vi "SetAutomaticParameterMode.vi"(7 "Auto Parameter":T2, 8 "error in (no error)":errorcluster, 10 "Automatic":T1, 11 "Stream in":refnum<class "Stream.lvclass">) -> (0 "error out":errorcluster, 3 "Stream (Duplicate)":refnum<class "Stream.lvclass">)   [LabVIEW 2020, in "g_ar_toolkit.capture.lvlib" / "Stream.lvclass"]
uses:
  Stream.lvclass
  Camera Automatic Parameters.ctl
  Camera Automatic Parameter Mode.ctl
  Stream.lvclass/Stream.ctl
  g_ar_toolkit.common/g_ar_toolkit.common.lvlib
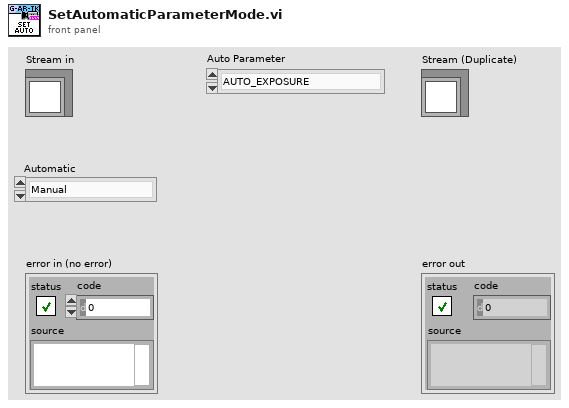
[diagram p1: front panel]
types:
  T1 = typedef "g_ar_toolkit.capture.lvlib/Stream.lvclass/Camera Automatic Parameter Mode.ctl" = enum16{"Manual", "Automatic"}
  T2 = typedef "g_ar_toolkit.capture.lvlib/Stream.lvclass/Camera Automatic Parameters.ctl" = enum16{"AUTO_EXPOSURE", "AUTO_FOCUS", "AUTO_WHITE_BALANCE", "AUTO_GAIN"}
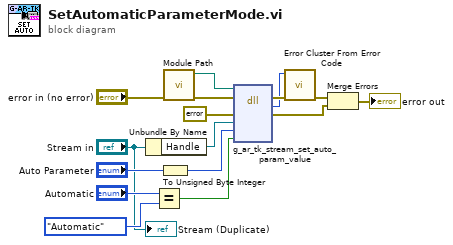
[diagram p0: block diagram]
diagram:
  n1 = Unbundle By Name("Stream in") -> ("Handle"=w13:refnum<data-value>)
  n2 = Equal?(x="Automatic", y=Camera_Automatic_Parameter_Mode."Automatic") -> (x = y?=w5:bool)
  n3 = To Unsigned Byte Integer(number="Auto Parameter") -> (unsigned 8bit integer=w7:u8)
  n4 = call "Module Path.vi"("error in (no error)"="error in (no error)") -> ("error out"=w2:errorcluster, "Path"=w1:path)  [unwired: 9 in]
  n5 = dll-call lib="?" fn="g_ar_tk_stream_set_auto_param_value" ("g_ar_toolkit.*.*:g_ar_tk_stream_capture_next")(path in=w1, error in=w2, "error_cluster"=errorcluster {"status"=FALSE, "code"=0, "source"=""} ("error constant"), "EDVR_strm"=w13, "parameter"=w7, "automatic"=w5) -> (error out=w12:errorcluster, "MgErr"=w11:i32, "error_cluster"=w9:errorcluster)  [unwired: 4 in, 1 out]
  n6 = call <vilib>:"Error Cluster From Error Code.vi"("error in (no error)"=w12, "error code (0)"=w11) -> ("error out"=w10:errorcluster)  [unwired: 7 in]
  n7 = Merge Errors(w10, w9) -> (→"error out":errorcluster)
  "Stream (Duplicate)" <- "Stream in"
